vi "Get_Initial_Displacements-2.vi"(3 "error IN":errorcluster, 4 "dR max":dbl, 5 "dR min":dbl, 6 "[IN] (X,Y)":dbl[][](array[numeric])) -> (0 "error OUT":errorcluster, 2 "[OUT] Raw Displacements":dbl[][](array[numeric]))   [LabVIEW 2013]
panel:
  out "# Displacements":i16
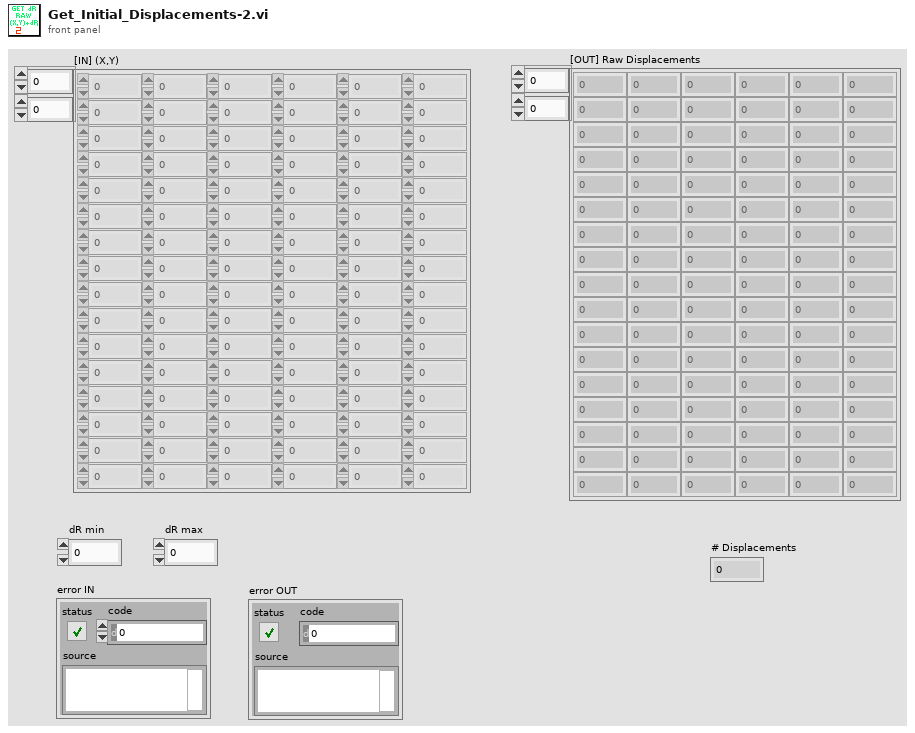
[diagram p1: front panel]
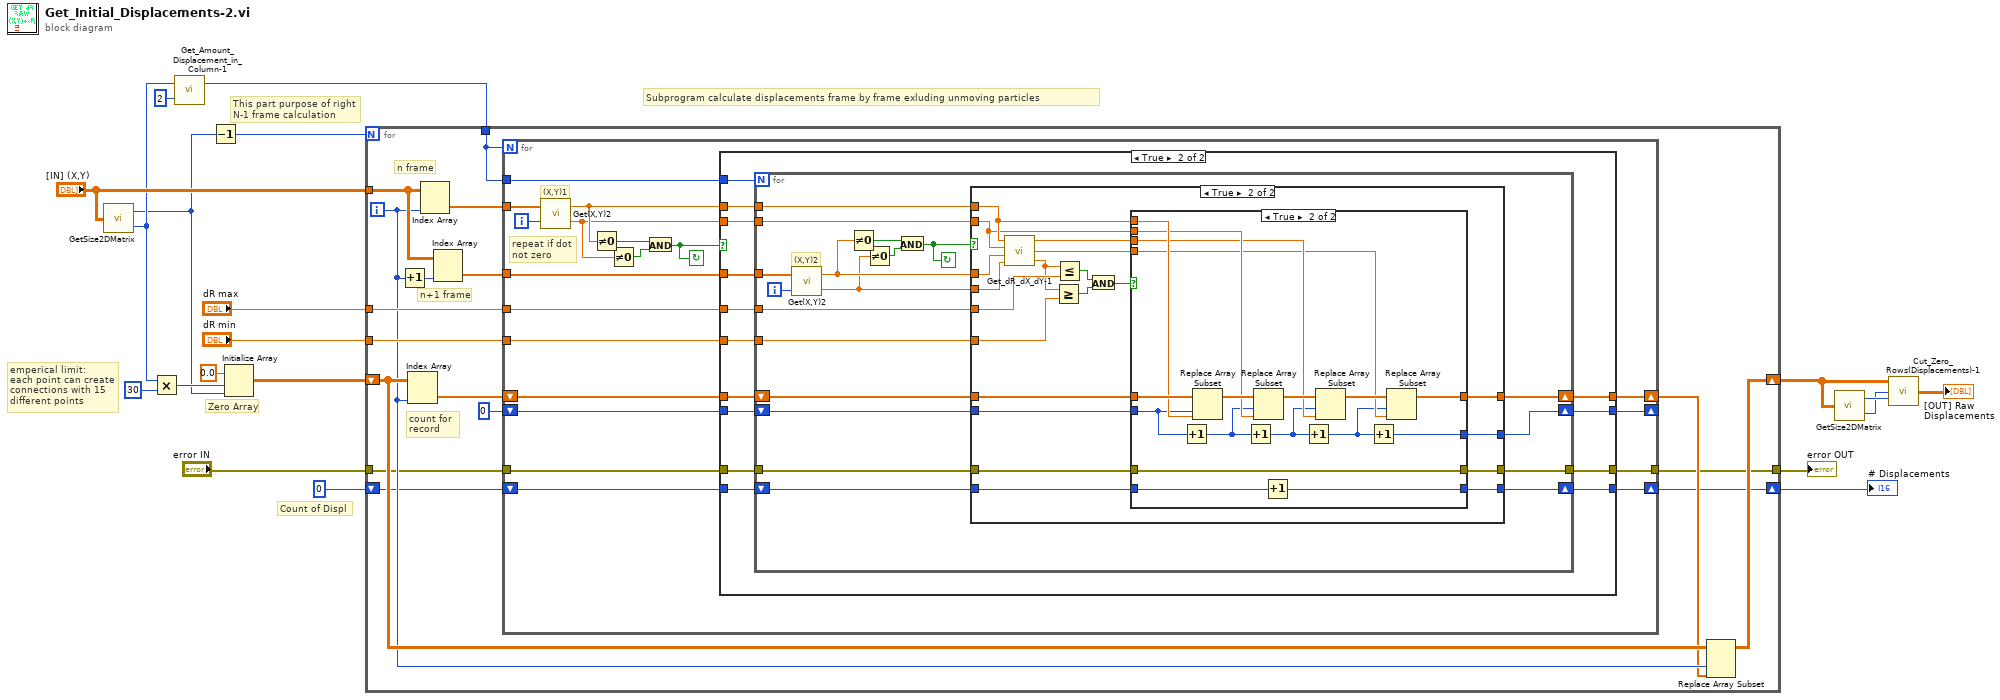
[diagram p0: block diagram]
diagram:
  # "emperical limit:\neach point can create \nconnections with 15 \ndifferent points"
  # "This part purpose of right\nN-1 frame calculation"
  # "Count of Displ"
  # "Subprogram calculate displacements frame by frame exluding unmoving particles"
  # "Zero Array"
  n1 = call "GetSize2DMatrix.vi"("Array IN (2D)"="[IN] (X,Y)") -> ("# Cols"=w2:i32, "# Rows"=w4:i32)
  n2 = Multiply(x=w4, y=30) -> (x*y=w18:i32)
  n3 = call "Get_Amount_Displacement_in_Column-1.vi"("multiplier"=2 ("y"), "# Rows"=w4) -> ("Displ amount"=w3:i32)  [unwired: 1 out]
  n4 = Decrement(x=w2) -> (x-1=w1:i32)
  n5 = Initialize Array(0.0 ("element"), w18, w2) -> (w16:dbl[][])
  n6 = for {
    N: w1 -> [_]
    tunnel: "[IN] (X,Y)" -> [w37]
    shift-right: [w26] -> w9
    shift-left: w16 -> [w29]
    tunnel: "dR max" -> [w33]
    tunnel: "dR min" -> [w32]
    tunnel: "error IN" -> [w25]
    tunnel: [w24] -> w12
    shift-right: [w22] -> w6
    shift-left: i16 0 -> [w23]
    tunnel: w3 -> [w21]
    i -> [w28]
    # "count for \nrecord"
    # "n+1 frame"
    # "n frame"
    n7 = Increment(x=w28) -> (x+1=w36:i32)
    n8 = Index Array(array=w29, index (col)=w28) -> (element=w31:dbl[])  [unwired: 1 in]
    n9 = Index Array(array=w37, index (col)=w28) -> (element=w35:dbl[])  [unwired: 1 in]
    n10 = Index Array(array=w37, index (col)=w36) -> (element=w34:dbl[])  [unwired: 1 in]
    n11 = for {
      N: w21 -> [_]
      tunnel: w35 -> [w44]
      tunnel: w21 -> [w56]
      tunnel: w34 -> [w55]
      tunnel: w33 -> [w54]
      tunnel: w32 -> [w53]
      shift-right: [w50] -> w27
      shift-left: w31 -> [w52]
      shift-right: [w49] -> _
      shift-left: 0 -> [w51]
      tunnel: w25 -> [w48]
      tunnel: [w47] -> w24
      shift-right: [w45] -> w22
      shift-left: w23 -> [w46]
      i -> [w43]
      stop <- w38 continue-if-true
      # "repeat if dot \nnot zero"
      # "(X,Y)1"
      n12 = call "Get(X,Y)2.vi"("[IN] index of (X,Y)"=w43, "[IN] Array coordi\nnates (X,Y) in Frame"=w44) -> ("[OUT] Y"=w41:dbl, "[OUT] X"=w42:dbl)
      n13 = Not Equal To 0?(x=w42) -> (x != 0?=w40:bool)
      n14 = Not Equal To 0?(x=w41) -> (x != 0?=w39:bool)
      n15 = And(x=w40, y=w39) -> (x .and. y?=w38:bool)
      n16 = case shown="True" w38 {
        tunnel: w56 -> [_ w74]
        tunnel: w55 -> [_ w73]
        tunnel: w54 -> [_ w72]
        tunnel: w53 -> [_ w71]
        tunnel: w52 -> [w60 w70]
        tunnel: w51 -> [w59 w69]
        tunnel: [w60 w68] -> w50
        tunnel: [w59 w67] -> w49
        tunnel: w48 -> [w58 w66]
        tunnel: [w58 w65] -> w47
        tunnel: w46 -> [w57 w64]
        tunnel: [w57 w63] -> w45
        tunnel: w42 -> [_ w62]
        tunnel: w41 -> [_ w61]
        frame False {
        }
        frame True {
          n17 = for {
            N: w74 -> [_]
            tunnel: w62 -> [w93]
            tunnel: w61 -> [w92]
            tunnel: w73 -> [w81]
            tunnel: w72 -> [w91]
            tunnel: w71 -> [w90]
            shift-right: [w86] -> w68
            shift-left: w70 -> [w89]
            shift-right: [w87] -> w67
            shift-left: w69 -> [w88]
            tunnel: w66 -> [w85]
            tunnel: [w84] -> w65
            shift-right: [w82] -> w63
            shift-left: w64 -> [w83]
            i -> [w80]
            stop <- w75 continue-if-true
            # "(X,Y)2"
            n18 = call "Get(X,Y)2.vi"("[IN] index of (X,Y)"=w80, "[IN] Array coordi\nnates (X,Y) in Frame"=w81) -> ("[OUT] Y"=w76:dbl, "[OUT] X"=w77:dbl)
            n19 = Not Equal To 0?(x=w77) -> (x != 0?=w79:bool)
            n20 = Not Equal To 0?(x=w76) -> (x != 0?=w78:bool)
            n21 = And(x=w79, y=w78) -> (x .and. y?=w75:bool)
            n22 = case shown="True" w75 {
              tunnel: w93 -> [_ w111]
              tunnel: w92 -> [_ w110]
              tunnel: w77 -> [_ w109]
              tunnel: w76 -> [_ w108]
              tunnel: w91 -> [_ w117]
              tunnel: w90 -> [_ w115]
              tunnel: w89 -> [w96 w107]
              tunnel: w88 -> [w97 w106]
              tunnel: [w97 w103] -> w87
              tunnel: [w96 w102] -> w86
              tunnel: w85 -> [w95 w101]
              tunnel: [w95 w100] -> w84
              tunnel: w83 -> [w94 w99]
              tunnel: [w94 w98] -> w82
              frame False {
              }
              frame True {
                n23 = call "Get_dR_dX_dY-1.vi"("Y2"=w108, "X2"=w109, "Y1"=w110, "X1"=w111) -> ("dR"=w116:dbl, "dY"=w104:dbl, "dX"=w105:dbl)
                n24 = Greater Or Equal?(x=w116, y=w115) -> (x >= y?=w113:bool)
                n25 = Less Or Equal?(x=w116, y=w117) -> (x <= y?=w114:bool)
                n26 = And(x=w114, y=w113) -> (x .and. y?=w112:bool)
                n27 = case shown="True" w112 {
                  tunnel: w111 -> [_ w137]
                  tunnel: w110 -> [_ w134]
                  tunnel: w107 -> [w120 w138]
                  tunnel: w106 -> [w121 w135]
                  tunnel: w105 -> [_ w131]
                  tunnel: w104 -> [_ w128]
                  tunnel: [w121 w126] -> w103
                  tunnel: [w120 w125] -> w102
                  tunnel: w101 -> [w119 w124]
                  tunnel: [w119 w124] -> w100
                  tunnel: w99 -> [w118 w123]
                  tunnel: [w118 w122] -> w98
                  frame False {
                  }
                  frame True {
                    n28 = Increment(x=w135) -> (x+1=w132:i32)
                    n29 = Replace Array Subset(array=w138, new element=w137, index=w135) -> (w136:dbl[])
                    n30 = Increment(x=w132) -> (x+1=w129:i32)
                    n31 = Replace Array Subset(array=w136, new element=w134, index=w132) -> (w133:dbl[])
                    n32 = Increment(x=w123) -> (x+1=w122:i16)
                    n33 = Increment(x=w129) -> (x+1=w127:i32)
                    n34 = Replace Array Subset(array=w133, new element=w131, index=w129) -> (w130:dbl[])
                    n35 = Increment(x=w127) -> (x+1=w126:i32)
                    n36 = Replace Array Subset(array=w130, new element=w128, index=w127) -> (w125:dbl[])
                  }
                }
              }
            }
          }
        }
      }
    }
    n37 = Replace Array Subset(array=w29, new element=w27, index (col)=w28) -> (w26:dbl[][])  [unwired: 1 in]
  }
  "error OUT" <- w12
  "# Displacements" <- w6
  n38 = call "GetSize2DMatrix.vi"("Array IN (2D)"=w9) -> ("# Cols"=w11:i32, "# Rows"=w10:i32)
  n39 = call "Cut_Zero_Rows(Displacements)-1.vi"("# Cols"=w11, "# Rows"=w10, "Array IN"=w9) -> ("Array OUT"=→"[OUT] Raw Displacements":dbl[][])
